vi "sub_UIupdate_T.vi"(8 "error in":errorcluster) -> (0 "error out":errorcluster)   [LabVIEW 2016]
uses:
  ctl/UI_cmd-ctl.ctl
  Global.vi
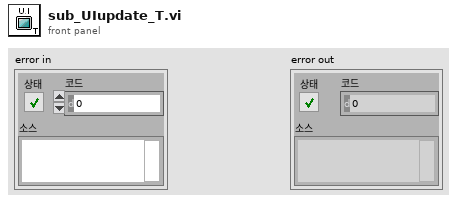
[diagram p1: front panel]
types:
  T1 = typedef "UI_cmd-ctl.ctl" = enum16{"default", "create", "read"}
  T2 = typedef "data.ctl" = cluster{"Bonding force":dbl, "Bonding time":dbl, "Bonding index":dbl, "Pickup force":dbl, "Pickup time":dbl, "Pickup index":dbl, "Detach force":dbl, "Detach time":dbl, "Detach index":dbl, "Heater temp rt":dbl, "Vacuum rt":dbl, "IR raw data":i16[][], "IR temp data":dbl[][], "vacuum raw wf":waveform(dbl), "vacuum kpa wf":waveform(dbl), "strain raw wf":waveform(dbl)[], "Force rt":dbl, "Vacuum T":dbl, "Heater temp T":dbl, "Balance xy arrays":cluster{dbl, dbl}[], "Balance xy":cluster{dbl, dbl}[], "Bonding wf index":dbl, "Pickup wf index":dbl, "Bonding rising index":dbl, "Bonding falling index":dbl, "Pickup rising index":dbl, "Pickup falling index":dbl}
  T3 = typedef "UI_ctl.ctl" = cluster{"Heater temp":refnum<vi>, "Heater chart":refnum<vi>, "vacuum (kpa)":refnum<vi>, "Balance xy graph":refnum<vi>, "Strain chart w cal":refnum<vi>, "Pickup force":refnum<vi>, "Pickup time":refnum<vi>, "Force chart":refnum<vi>, "Force graph T":refnum<vi>, "vacuum chart":refnum<vi>, "vacuum rt":refnum<vi>, "Strain raw graph":refnum<vi>, "Strain raw chart":refnum<vi>, "Bonding time":refnum<vi>, "Bonding force":refnum<vi>, "Balance":refnum<vi>, "Filtered force graph":refnum<vi>, "ROI intensity":refnum<vi>, "Heater_rt":refnum<vi>, "Detach force":refnum<vi>, "Force rt":refnum<vi>, "Mixed signal":refnum<vi>}
  T4 = cluster{"PCB temp":refnum<vi>, "Vacuum":refnum<vi>, "PCB config":refnum<vi>, "Balance_x":refnum<vi>, "Balance_y":refnum<vi>}
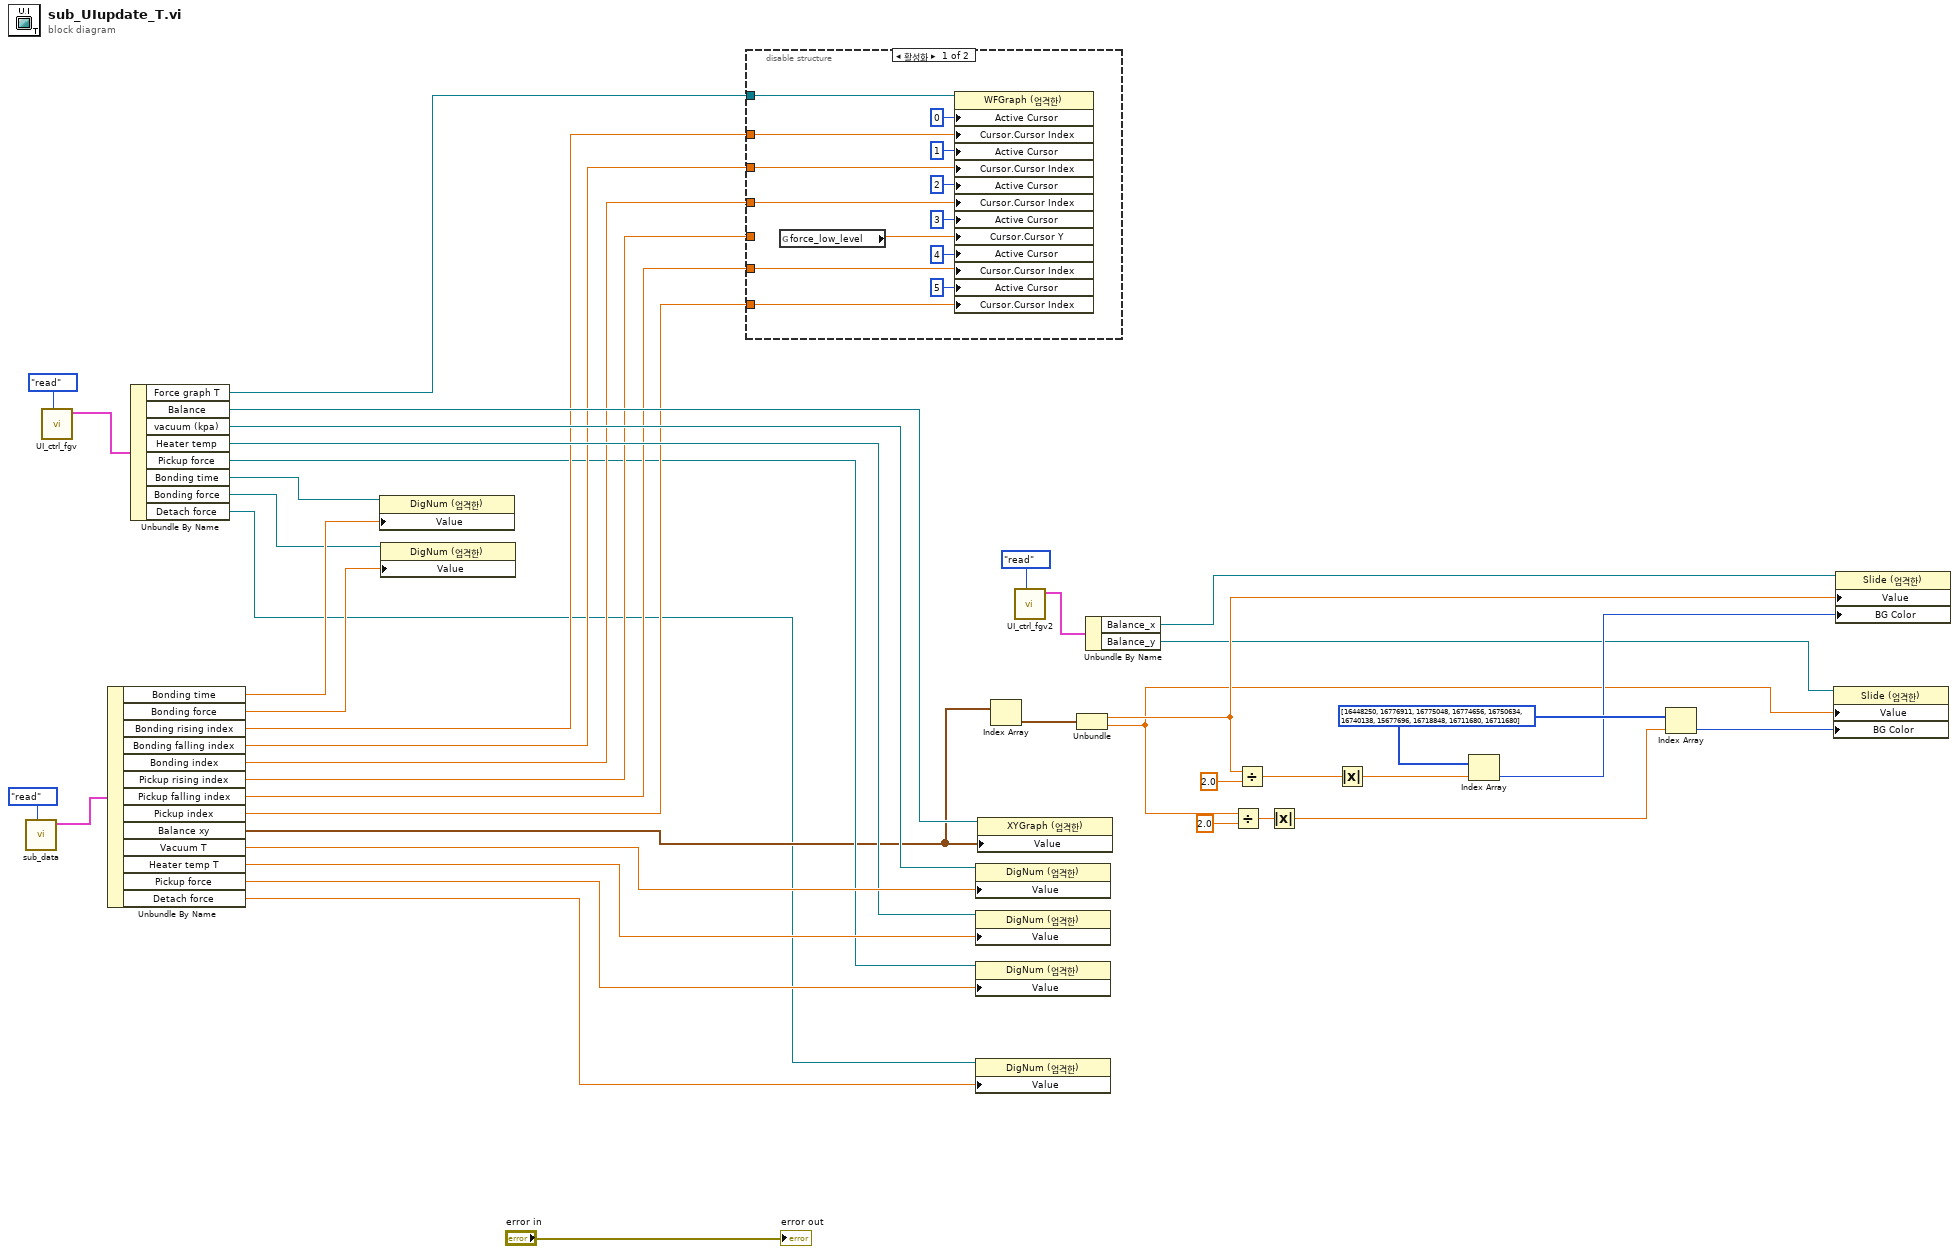
[diagram p0: block diagram]
diagram:
  w20 = u32[] [16448250, 16776911, 16775048, 16774656, 16750634, 16740138, 15677696, 16718848, 16711680, 16711680]
  n1 = call "sub_data.vi"("cmd"=enum16{"ini", "write", "read"}."read") -> ("data out"=w38:T2)  [unwired: 9 in, 1 out]
  n2 = call "UI_ctrl_fgv.vi"("cmd"=UI_cmd-ctl."read") -> ("UI cluster out"=w39:T3)  [unwired: 10 in]
  n3 = Unbundle By Name(w38) -> ("Bonding time"=w5:dbl, "Bonding force"=w3:dbl, "Bonding rising index"=w31:dbl, "Bonding falling index"=w30:dbl, "Bonding index"=w29:dbl, "Pickup rising index"=w28:dbl, "Pickup falling index"=w27:dbl, "Pickup index"=w26:dbl, "Balance xy"=w23:cluster{dbl, dbl}[], "Vacuum T"=w35:dbl, "Heater temp T"=w33:dbl, "Pickup force"=w24:dbl, "Detach force"=w2:dbl)
  n4 = Unbundle By Name(w39) -> ("Force graph T"=w32:refnum<vi>, "Balance"=w37:refnum<vi>, "vacuum (kpa)"=w36:refnum<vi>, "Heater temp"=w34:refnum<vi>, "Pickup force"=w25:refnum<vi>, "Bonding time"=w6:refnum<vi>, "Bonding force"=w4:refnum<vi>, "Detach force"=w1:refnum<vi>)
  n5 = property class="DigNum (엄격한)"(reference=w6, "Value"=w5) -> ()  [unwired: 1 in, 2 out]
  n6 = property class="DigNum (엄격한)"(reference=w4, "Value"=w3) -> ()  [unwired: 1 in, 2 out]
  n7 = disable-structure shown="활성화" {
    disable-tunnel: w32 -> [w55 _]
    disable-tunnel: w31 -> [w48 _]
    disable-tunnel: w30 -> [w47 _]
    disable-tunnel: w29 -> [w46 _]
    disable-tunnel: w28 -> [_ _]
    disable-tunnel: w27 -> [w45 _]
    disable-tunnel: w26 -> [w44 _]
    frame Enabled {
      n8 = global read "Global.vi" "force_low_level"() -> (w43:dbl)
      n9 = property class="WFGraph (엄격한)"(reference=w55, "Active Cursor"=u32 0 ("활성 커서"), "Cursor.Cursor Index"=w48, "Active Cursor"=u32 1 ("활성 커서"), "Cursor.Cursor Index"=w47, "Active Cursor"=u32 2 ("활성 커서"), "Cursor.Cursor Index"=w46, "Active Cursor"=u32 3 ("활성 커서"), "Cursor.Cursor Y"=w43, "Active Cursor"=u32 4 ("활성 커서"), "Cursor.Cursor Index"=w45, "Active Cursor"=u32 5 ("활성 커서"), "Cursor.Cursor Index"=w44) -> ()  [unwired: 1 in, 2 out]
    }
    frame Disabled {
    }
  }
  n10 = property class="DigNum (엄격한)"(reference=w36, "Value"=w35) -> ()  [unwired: 1 in, 2 out]
  n11 = property class="DigNum (엄격한)"(reference=w34, "Value"=w33) -> ()  [unwired: 1 in, 2 out]
  n12 = property class="DigNum (엄격한)"(reference=w25, "Value"=w24) -> ()  [unwired: 1 in, 2 out]
  n13 = property class="DigNum (엄격한)"(reference=w1, "Value"=w2) -> ()  [unwired: 1 in, 2 out]
  n14 = property class="XYGraph (엄격한)"(reference=w37, "Value"=w23) -> ()  [unwired: 1 in, 2 out]
  n15 = Index Array(array=w23) -> (element=w16:cluster{dbl, dbl})  [unwired: 1 in]
  n16 = call "UI_ctrl_fgv2.vi"("cmd"=enum16{"read", "create"}."read") -> ("UI out"=w21:T4)  [unwired: 10 in]
  n17 = Unbundle(w16) -> (w11:dbl, w8:dbl)
  n18 = Unbundle By Name(w21) -> ("Balance_x"=w12:refnum<vi>, "Balance_y"=w9:refnum<vi>)
  n19 = Divide(x=w8, y=2.0) -> (x/y=w14:dbl)
  n20 = Divide(x=w11, y=2.0) -> (x/y=w18:dbl)
  n21 = Absolute Value(x=w14) -> (abs(x)=w13:dbl)
  n22 = Absolute Value(x=w18) -> (abs(x)=w19:dbl)
  n23 = Index Array(array=w20, index=w19) -> (element=w10:u32)
  n24 = Index Array(array=w20, index=w13) -> (element=w7:u32)
  n25 = property class="Slide (엄격한)"(reference=w9, "Value"=w8, "BG Color"=w7) -> ()  [unwired: 1 in, 2 out]
  n26 = property class="Slide (엄격한)"(reference=w12, "Value"=w11, "BG Color"=w10) -> ()  [unwired: 1 in, 2 out]
  "error out" <- "error in"
